vi "basic usage.vi"() -> ()   [LabVIEW 2016]
uses:
  API/JSON Document Class/json insert/json Insert - String Path.vi
  API/JSON Document Class/json to string/json To Minimized String - string path.vi
  API/JSON Document Class/json parse/poly instances/json Parse I32 - string path.vi
  API/JSON Document Class/json parse/poly instances/json Parse String - string path.vi
  API/JSON Document Class/json delete/json Delete - string path.vi
  API/JSON Document Class/JSON Document.lvclass
panel:
  in  "error in (no error)":errorcluster
  out "error out":errorcluster
  out "removing keys":string
  out "defaulted?":bool
  out "defaulting values":string
  out "automatically generating parents":string
  out "modifying values":string
  out "adding keys":string
  # "This VI shows basic usage of the API, including adding values to a JSON Document, modifying values, and removing them."
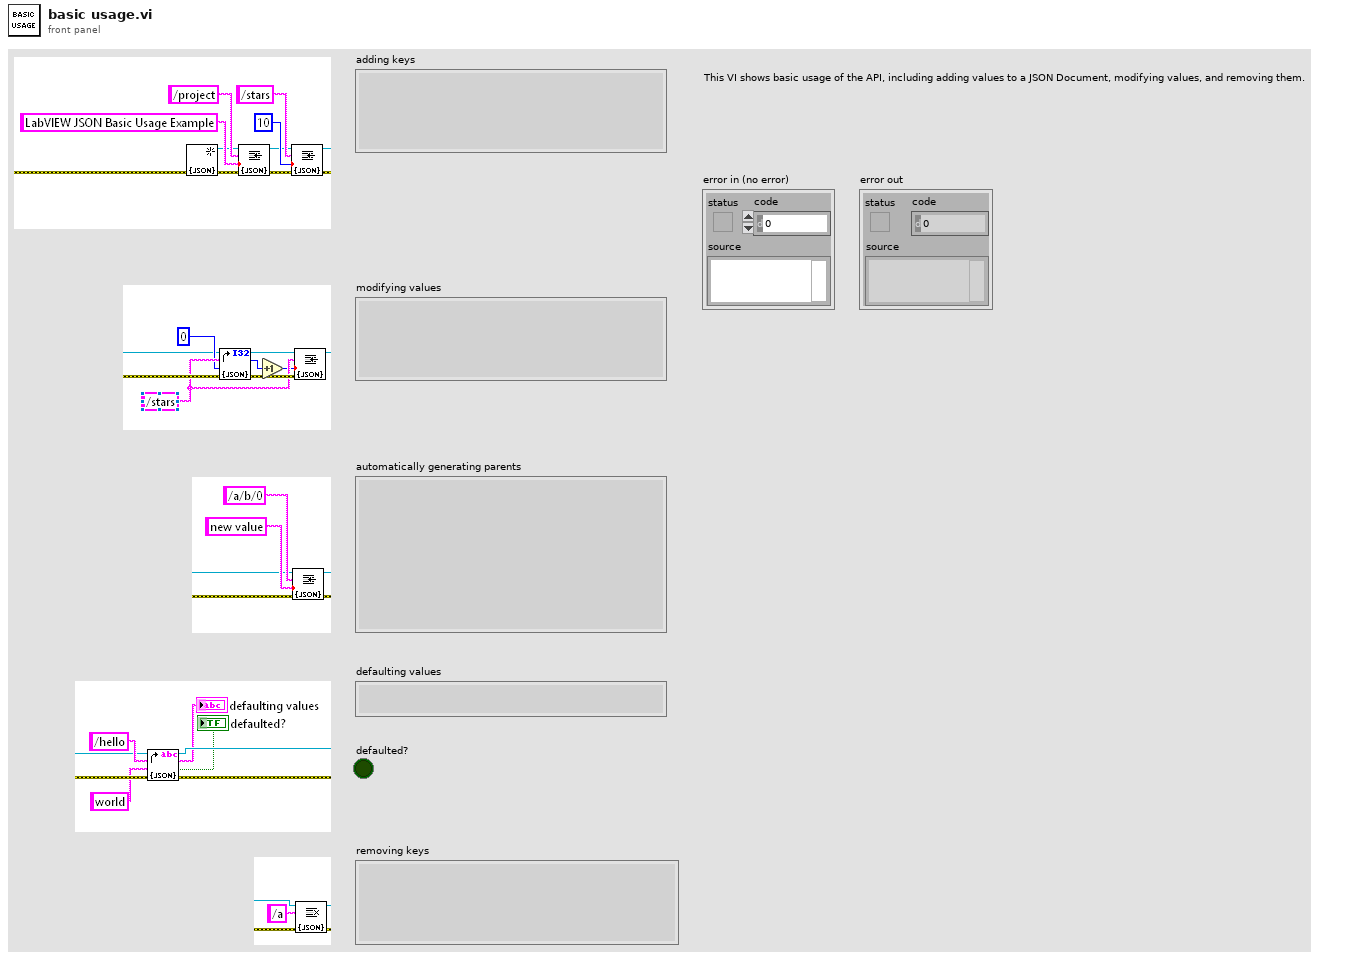
[diagram p1: front panel]
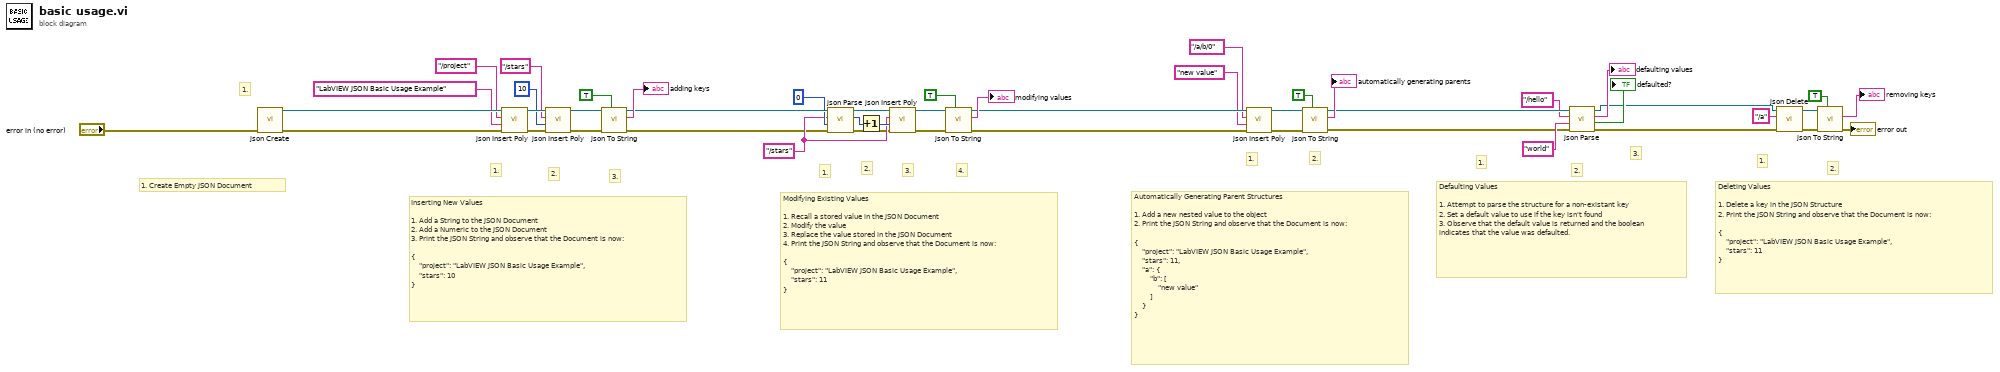
[diagram p0: block diagram]
diagram:
  w19 = "/stars" ("path")
  # "2."
  # "1."
  # "3."
  # "2."
  # "1."
  # "2."
  # "1."
  # "4."
  # "3."
  # "2."
  # "1."
  # "3."
  # "2."
  # "1."
  # "1."
  # "Deleting Values\n\n1. Delete a key in the JSON Structure\n2. Print the JSON String and observe that the Document is now:\n\n{\n    \"project\": \"LabVIEW JSON Basic Usage Example\",\n    \"stars\": 11\n}"
  # "Defaulting Values\n\n1. Attempt to parse the structure for a non-existant key\n2. Set a default value to use if the key isn't found\n3. Observe that the default value is returned and the boolean indicates that the value was defaulted."
  # "Automatically Generating Parent Structures\n\n1. Add a new nested value to the object\n2. Print the JSON String and observe that the Document is now:\n\n{\n    \"project\": \"LabVIEW JSON Basic Usage Example\",\n    \"stars\": 11,\n    \"a\": {\n        \"b\": [\n            \"new value\"\n        ]\n    }\n}"
  # "Modifying Existing Values\n\n1. Recall a stored value in the JSON Document\n2. Modify the value\n3. Replace the value stored in the JSON Document\n4. Print the JSON String and observe that the Document is now:\n\n{\n    \"project\": \"LabVIEW JSON Basic Usage Example\",\n    \"stars\": 11\n}"
  # "Inserting New Values\n\n1. Add a String to the JSON Document\n2. Add a Numeric to the JSON Document\n3. Print the JSON String and observe that the Document is now:\n\n{\n    \"project\": \"LabVIEW JSON Basic Usage Example\",\n    \"stars\": 10\n}"
  # "1. Create Empty JSON Document"
  n1 = call "json Create.vi"("error in (no error)"="error in (no error)") -> ("error out"=w46:errorcluster, "JSON Document out"=w47:refnum<class "JSON Document.lvclass">)  [unwired: 9 in]
  n2 = call-poly "json Insert Poly.vi"("error in (no error)"=w46, "anything"="LabVIEW JSON Basic Usage Example" ("path"), "path"="/project", "JSON Document in"=w47) -> ("error out"=w43:errorcluster, "JSON Document out"=w42:refnum<class "JSON Document.lvclass">)  [unwired: 5 in, 1 out]
  n3 = call-poly "json Insert Poly.vi"("error in (no error)"=w43, "anything"=10, "path"="/stars", "JSON Document in"=w42) -> ("error out"=w35:errorcluster, "JSON Document out"=w38:refnum<class "JSON Document.lvclass">)  [unwired: 5 in, 1 out]
  n4 = call-poly "json To String.vi"("pretty print?"=TRUE, "error in (no error)"=w35, "JSON Document in"=w38) -> ("error out"=w4:errorcluster, "json string"=→"adding keys":string, "JSON Document out"=w21:refnum<class "JSON Document.lvclass">)  [unwired: 6 in]
  n5 = call-poly "json Parse.vi"("error in (no error)"=w4, "default"=0, "path"=w19, "JSON Document in"=w21) -> ("error out"=w2:errorcluster, "value"=w18:i32, "JSON Document out"=w22:refnum<class "JSON Document.lvclass">)  [unwired: 4 in, 1 out]
  n6 = Increment(x=w18) -> (x+1=w39:i32)
  n7 = call-poly "json Insert Poly.vi"("error in (no error)"=w2, "anything"=w39, "path"=w19, "JSON Document in"=w22) -> ("error out"=w34:errorcluster, "JSON Document out"=w33:refnum<class "JSON Document.lvclass">)  [unwired: 5 in, 1 out]
  n8 = call-poly "json To String.vi"("pretty print?"=TRUE, "error in (no error)"=w34, "JSON Document in"=w33) -> ("error out"=w30:errorcluster, "json string"=→"modifying values":string, "JSON Document out"=w29:refnum<class "JSON Document.lvclass">)  [unwired: 6 in]
  n9 = call-poly "json Insert Poly.vi"("error in (no error)"=w30, "anything"="new value", "path"="/a/b/0", "JSON Document in"=w29) -> ("error out"=w26:errorcluster, "JSON Document out"=w25:refnum<class "JSON Document.lvclass">)  [unwired: 5 in, 1 out]
  n10 = call-poly "json To String.vi"("pretty print?"=TRUE, "error in (no error)"=w26, "JSON Document in"=w25) -> ("error out"=w12:errorcluster, "json string"=→"automatically generating parents":string, "JSON Document out"=w17:refnum<class "JSON Document.lvclass">)  [unwired: 6 in]
  n11 = call-poly "json Parse.vi"("error in (no error)"=w12, "default"="world", "path"="/hello", "JSON Document in"=w17) -> ("error out"=w10:errorcluster, "defaulted?"=→"defaulted?":bool, "value"=→"defaulting values":string, "JSON Document out"=w11:refnum<class "JSON Document.lvclass">)  [unwired: 4 in]
  n12 = call-poly "json Delete.vi"("error in (no error)"=w10, "path"="/a", "JSON Document in"=w11) -> ("error out"=w8:errorcluster, "JSON Document out"=w7:refnum<class "JSON Document.lvclass">)  [unwired: 6 in, 1 out]
  n13 = call-poly "json To String.vi"("pretty print?"=TRUE, "error in (no error)"=w8, "JSON Document in"=w7) -> ("error out"=→"error out":errorcluster, "json string"=→"removing keys":string)  [unwired: 6 in, 1 out]
